vi "Get Next Transfer Size.vi"(0 "disk streaming in":refnum<class "Disk Streaming.lvclass">, 5 "error in (no error)":errorcluster) -> (14 "disk streaming out":refnum<class "Disk Streaming.lvclass">, 15 "elements to transfer":u32, 19 "error out":errorcluster)   [LabVIEW 2021, in "Disk Streaming.lvclass"]
doc: "Returns the number of elements to transfer in the next block of a streaming process controlled by a disk streaming instance. For more information about the disk streaming instance refer to the <B>Open.vi</B> context help.\n\nInputs:\n\n<B>disk streaming in</B>: Disk streaming instance input.\n\nOutputs:\n\n<B>disk streaming out</B>: Disk streaming instance output. Pass this output to the other Disk Streaming VIs to perform the streaming.\n\n<B>elements to transfer</B>: The number of elements to transfer in the next block of the streaming process. A return value of zero signals that the streaming process is complete."
uses:
  Disk Streaming.lvclass
  Disk Streaming.lvclass/Disk Streaming.ctl
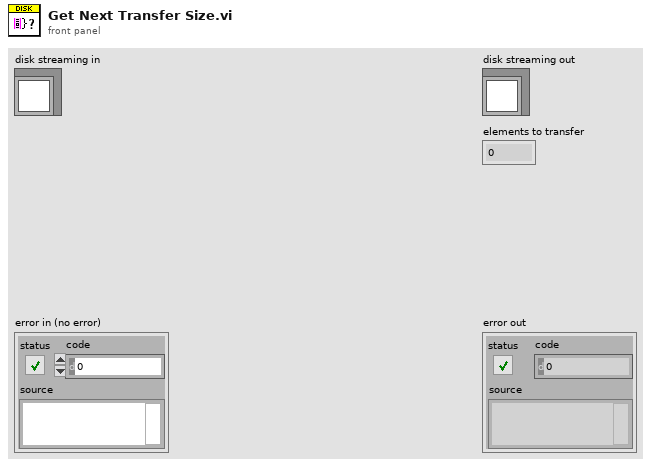
[diagram p1: front panel]
types:
  T1 = typedef "Disk Streaming.lvclass/Data.ctl" = cluster{"tdms file":refnum<k34>, "group name":string, "channel name":string, "max operations":u32, "timeout (s)":dbl, "data type size (bytes)":u64, "writing":bool, "I/O mode":T2, "# of blocks":u32, "block size divisor (bytes)":u32, "file position (elements)":u64, "file size (elements)":i64, "file size (samples)":i64, "block size (elements)":u64, "block size (samples)":u64, "quantum size (elements)":u64, "quantum size (samples)":u64, "samples remaining":i64, "elements transferred":u64, "finished":bool, "preview size":i32, "preview quantum size (elements)":u64, "preview quantum size (samples)":u64, "DMA buffer size (elements)":u32, "pending block sizes (bytes)":u64[]}
  T2 = typedef "Disk Streaming.lvclass/IO mode.ctl" = enum16{"Synchronous", "Asynchronous", "Data Reference"}
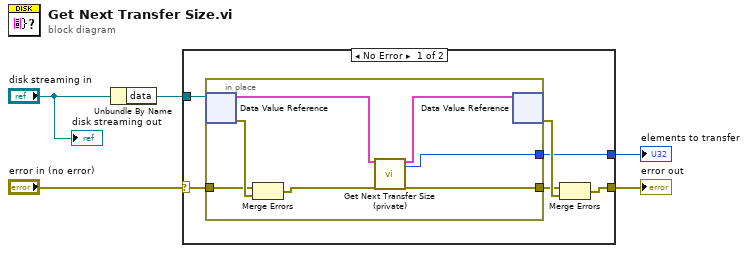
[diagram p0: block diagram]
diagram:
  n1 = Unbundle By Name("disk streaming in") -> ("data"=w1:refnum<data-value>)
  n2 = case shown="No Error" "error in (no error)" {
    selector: "error in (no error)" -> [w10 w19]
    tunnel: [w9 w19] -> w4
    tunnel: w1 -> [w8 _]
    tunnel: [w6 _] -> w3
    frame No Error {
      n3 = in-place {
        in-place-border: w10 -> [w17]
        in-place-border: [w15] -> w7
        in-place-border: [w12] -> w6
        n4 = in-place-dvr #1(w8) -> (w14:T1, w18:errorcluster)
        n5 = Merge Errors(w17, w18) -> (w16:errorcluster)
        n6 = call "Get Next Transfer Size (private).vi"("data in"=w14, "error in (no error)"=w16) -> ("data out"=w13:T1, "elements to transfer"=w12:u32, "error out"=w15:errorcluster)  [unwired: 15 in]
        n7 = in-place-dvr #1(w13) -> (w11:errorcluster)  [unwired: 1 out]
      }
      n8 = Merge Errors(w7, w11) -> (w9:errorcluster)
    }
    frame Error {
    }
  }
  "error out" <- w4
  "elements to transfer" <- w3
  "disk streaming out" <- "disk streaming in"
